vi "FarfiledImageJoint2.vi"() -> (1 "远场图像":T1(plugin-control))   [LabVIEW 2018]
uses:
  Init/AllPath.vi
  <vilib>/vision/NI_Vision_Development_Module.lvlib
panel:
  in  "停止":bool
  out "进度":dbl format="%05.2f%"
  out "俯仰":dbl
  out "Y Resolution":i32
  out "X Resolution":i32
  out "运行总时间s":dbl
  out "单步总时间ms":u32
  out "时间":u32[](array[numeric])
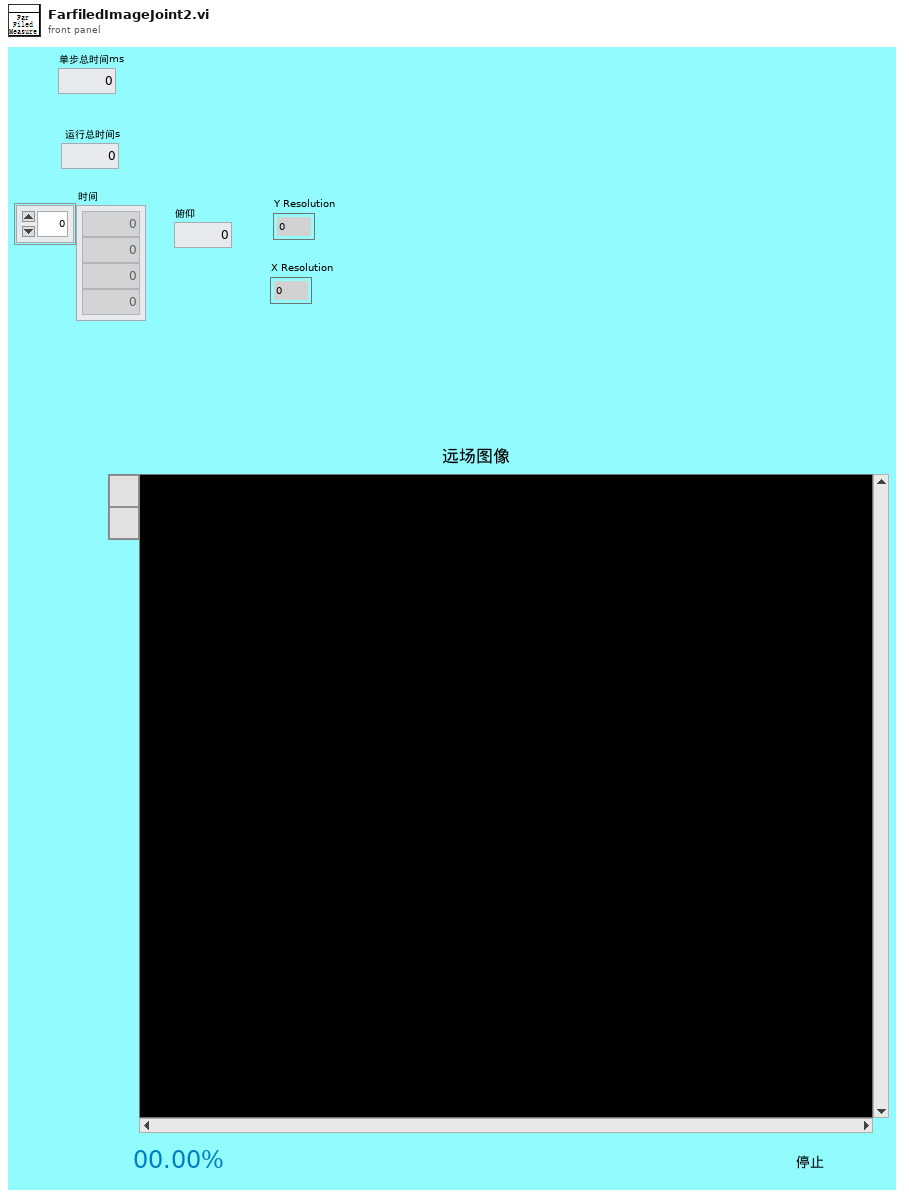
[diagram p1: front panel]
types:
  T1 = typedef "IMAQ Image.ctl" = refnum<image>
  T2 = typedef "Image Type" = u32
  T3 = typedef "控制电机枚举器.ctl" = enum16{"Z", "Y", "X", "发散角", "俯仰", "旋转"}
  T4 = cluster{"远场相机":cluster{"控制电机":T3, "位置":dbl}[], "近场相机":cluster{"控制电机":T3, "位置":dbl}[], "时间波形":cluster{"控制电机":T3, "位置":dbl}[], "偏振":cluster{"控制电机":T3, "位置":dbl}[], "能量":cluster{"控制电机":T3, "位置":dbl}[], "功率":cluster{"控制电机":T3, "位置":dbl}[], "光谱":cluster{"控制电机":T3, "位置":dbl}[], "准直光焦点":cluster{"控制电机":T3, "位置":dbl}[]}
  T5 = cluster{"能量/功率":path, " 示波器":path, " 光谱仪":path, "偏振":path, "近远场":cluster{" 近场图片":path, " 远场图片":path, "发散角数据":path}, "参数":path, " 基路径":path, "文件名信息":path, "输出模板路径":path, "输出报告路径":path}
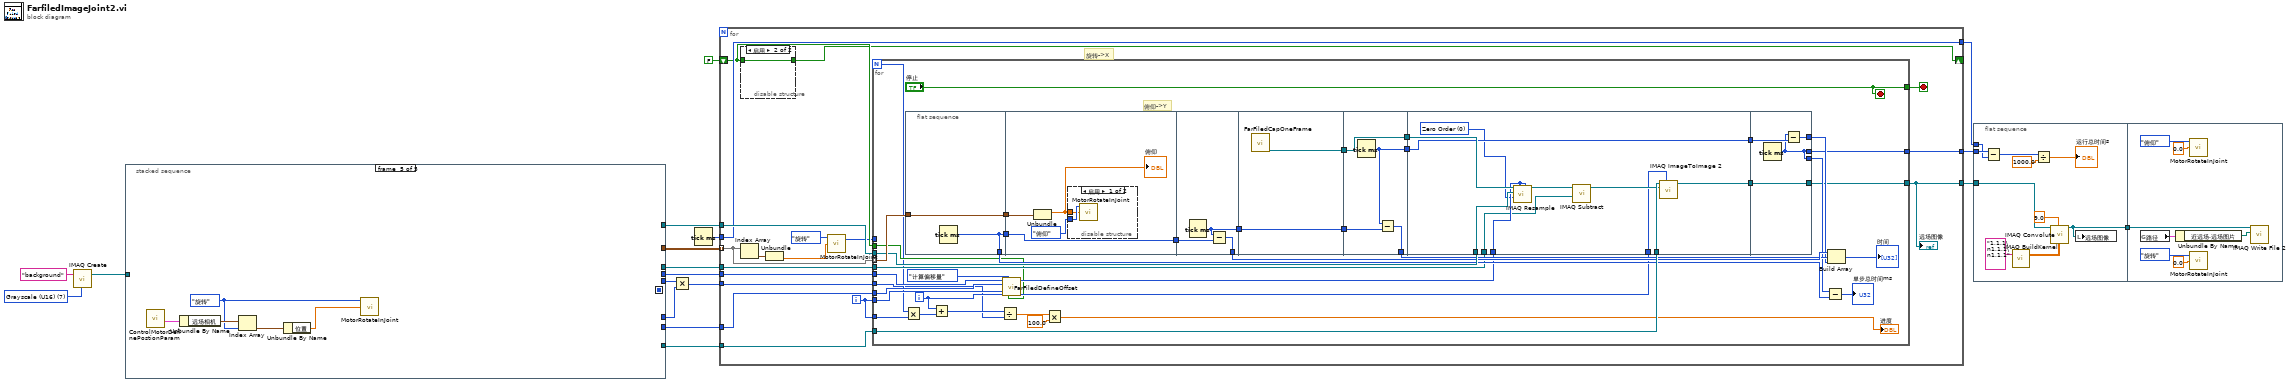
[diagram p0: block diagram]
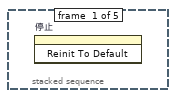
[diagram p2: hidden frame]
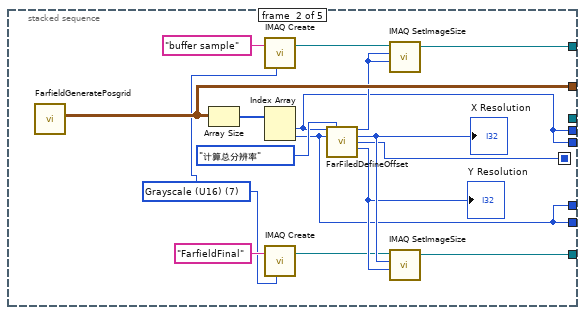
[diagram p3: hidden frame]
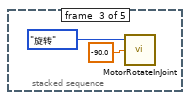
[diagram p4: hidden frame]
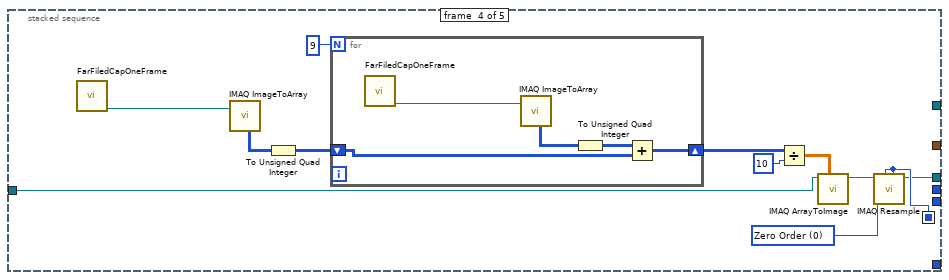
[diagram p5: hidden frame]
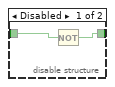
[diagram p6: hidden frame]
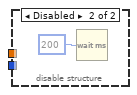
[diagram p7: hidden frame]
diagram:
  w1 = T2 7 items=["Grayscale (U8)", "Grayscale (I16)", "Grayscale (SGL)", "Complex (CSG)", "RGB (U32)", "HSL (U32)", "RGB (U64)", "Grayscale (U16)"] ("Image Type")
  n1 = call "IMAQ Create"("Image Name"="background", "Image Type"=w1) -> ("New Image"=w3:T1)  [unwired: 3 in, 1 out]
  n2 = stacked-sequence {
    seq-local: [_ w19 _ _ _] -> [_ _ _ w39 _]
    tunnel: [_ w34 _ _ _] -> w18
    tunnel: [_ w29 _ _ _] -> w17
    tunnel: [_ w28 _ _ _] -> w16
    tunnel: [_ w21 _ _ _] -> w15
    tunnel: [_ w22 _ _ _] -> w13
    tunnel: [_ _ _ w38 _] -> w9
    tunnel: [_ w22 _ _ _] -> w7
    tunnel: [_ w21 _ _ _] -> w6
    tunnel: w3 -> [_ _ _ w41 _]
    frame #0 {
      n3 = invoke on="停止" class="Bool" method="Reinit To Default"() -> ()  [unwired: 3 in, 3 out]
    }
    frame #1 {
      w26 = T2 7 items=["Grayscale (U8)", "Grayscale (I16)", "Grayscale (SGL)", "Complex (CSG)", "RGB (U32)", "HSL (U32)", "RGB (U64)", "Grayscale (U16)"] ("Image Type")
      n4 = call "FarfieldGeneratePosgrid.vi"() -> ("posOut"=w34:cluster{"俯仰":dbl, "旋转":dbl}[][])  [unwired: 9 in, 2 out]
      n5 = Array Size(array=w34) -> (size(s)=w33:i32[])
      n6 = call "IMAQ Create"("Image Name"="buffer sample", "Image Type"=w26) -> ("New Image"=w30:T1)  [unwired: 3 in, 1 out]
      n7 = Index Array(array=w33) -> (element #1=w22:i32, element #2=w21:i32)  [unwired: 2 in]
      n8 = call "IMAQ Create"("Image Name"="FarfieldFinal", "Image Type"=w26) -> ("New Image"=w20:T1)  [unwired: 3 in, 1 out]
      n9 = call "FarFiledDefineOffset.vi"("X Pos Num"=w22, "状态"=enum16{"计算总分辨率", "计算偏移量"}."计算总分辨率", "Y Pos Num"=w21) -> ("单个分辨率X"=w23:i32, "X Resolution"=w25:i32, "单个分辨率Y"=w19:i32, "Y Resolution"=w24:i32)  [unwired: 8 in, 1 out]
      "X Resolution" <- w25
      "Y Resolution" <- w24
      n10 = call "IMAQ SetImageSize"("Y Resolution"=w23, "X Resolution"=w23, "Image"=w30) -> ("Image Out"=w29:T1)  [unwired: 2 in, 1 out]
      n11 = call "IMAQ SetImageSize"("Y Resolution"=w24, "X Resolution"=w25, "Image"=w20) -> ("Image Out"=w28:T1)  [unwired: 2 in, 1 out]
    }
    frame #2 {
      n12 = call "MotorRotateInJoint.vi"("位置"=-90.0, "axis"=控制电机枚举器."旋转" ("控制电机")) -> ()  [unwired: 2 in, 1 out]
    }
    frame #3 {
      w37 = u32 0 items=["Zero Order", "Bi-Linear", "Quadratic", "Cubic Spline"] ("Interpolation Type")
      n13 = call "FarFiledCapOneFrame.vi"() -> ("Image_Normal"=w47:T1)  [unwired: 11 in]
      n14 = call "IMAQ ImageToArray"("Image"=w47) -> ("Image Pixels (U16)"=w45:u16[][])  [unwired: 3 in, 4 out]
      n15 = To Unsigned Quad Integer(1:w45) -> (0:w46:u64[][])
      n16 = for {
        N: 9 -> [_]
        shift-right: [w51] -> w44
        shift-left: w46 -> [w52]
        n17 = call "FarFiledCapOneFrame.vi"() -> ("Image_Normal"=w53:T1)  [unwired: 11 in]
        n18 = call "IMAQ ImageToArray"("Image"=w53) -> ("Image Pixels (U16)"=w50:u16[][])  [unwired: 3 in, 4 out]
        n19 = To Unsigned Quad Integer(1:w50) -> (0:w49:u64[][])
        n20 = Add(x=w49, y=w52) -> (x+y=w51:u64[][])
      }
      n21 = Divide(x=w44, y=10) -> (x/y=w42:dbl[][])
      n22 = call "IMAQ ArrayToImage"("Image Pixels (U16)"=w42, "Image"=w41) -> ("Image Out"=w40:T1)  [unwired: 8 in, 1 out]
      n23 = call "IMAQ Resample"("X Resolution"=w39, "Y Resolution"=w39, "Interpolation Type"=w37, "Image Src"=w40) -> ("Image Dst Out"=w38:T1)  [unwired: 6 in, 1 out]
    }
    frame #4 {
      w56 = 控制电机枚举器."旋转" ("控制电机")
      n24 = call "ControlMotorDefinePostionParam.vi"() -> ("位置信息"=w58:T4)  [unwired: 11 in]
      n25 = Unbundle By Name(w58) -> ("远场相机"=w57:cluster{"控制电机":T3, "位置":dbl}[])
      n26 = Index Array(array=w57, index=w56) -> (element=w55:cluster{"控制电机":T3, "位置":dbl})
      n27 = Unbundle By Name(w55) -> ("位置"=w54:dbl)
      n28 = call "MotorRotateInJoint.vi"("位置"=w54, "axis"=w56) -> ()  [unwired: 2 in, 1 out]
    }
  }
  n29 = Multiply(x=w7, y=w6) -> (x*y=w5:i32)
  n30 = Tick Count (ms)() -> (millisecond timer value=w12:u32)
  n31 = for "For循环" {
    tunnel: w18 -> [w72] mode=indexing
    tunnel: w17 -> [w76]
    tunnel: w13 -> [w74]
    tunnel: w15 -> [w73]
    shift-right: [w65] -> _
    shift-left: FALSE -> [w66]
    tunnel: w16 -> [w75]
    tunnel: [w62] -> w8
    tunnel: w12 -> [w67]
    tunnel: [w68] -> w11
    tunnel: [w67] -> w10
    tunnel: w9 -> [w64]
    tunnel: w5 -> [w59]
    i -> [w60]
    stop <- w61 stop-if-true
    # "旋转->X"
    n32 = disable-structure shown="启用" {
      disable-tunnel: w66 -> [w78 w79]
      disable-tunnel: [w77 w79] -> w65
      frame Disabled {
        n33 = Not(x=w78) -> (.not. x?=w77:bool)
      }
      frame Enabled {
      }
    }
    n34 = Index Array(array=w72) -> (element=w71:cluster{"俯仰":dbl, "旋转":dbl})  [unwired: 1 in]
    n35 = Unbundle(w71) -> ("旋转"=w69:dbl)  [unwired: 1 out]
    n36 = call "MotorRotateInJoint.vi"("位置"=w69, "axis"=控制电机枚举器."旋转" ("控制电机")) -> ("返回"=w63:i32)  [unwired: 2 in]
    n37 = for "For循环" {
      N -> [w84]
      tunnel: w72 -> [w119] mode=indexing
      tunnel: w76 -> [w118]
      tunnel: w60 -> [w97]
      tunnel: w74 -> [w95]
      tunnel: w73 -> [w96]
      tunnel: w66 -> [w92]
      tunnel: w75 -> [w117]
      tunnel: [w90] -> w62
      tunnel: [w100] -> w68
      tunnel: w64 -> [w99]
      tunnel: w63 -> [_]
      tunnel: ["停止"] -> w61
      tunnel: w60 -> [w85]
      tunnel: w59 -> [w83]
      i -> [w86]
      stop <- "停止" stop-if-true
      # "俯仰->Y"
      n38 = Multiply(x=w84, y=w85) -> (x*y=w88:i32)
      n39 = flat-sequence {
        tunnel: w119 -> [w121]
        tunnel: [w121] -> w112
        tunnel: [w120] -> w111
        tunnel: [w120] -> w102
        tunnel: w112 -> [w124]
        tunnel: w111 -> [w125]
        tunnel: [w125] -> w91
        tunnel: [w131] -> w110
        tunnel: w91 -> [w130]
        tunnel: [w129] -> w116
        tunnel: [w132] -> w109
        tunnel: w110 -> [w133]
        tunnel: [w133] -> w108
        tunnel: w109 -> [w137]
        tunnel: [w137] -> w107
        tunnel: [w135] -> w106
        tunnel: w108 -> [w136]
        tunnel: [w134] -> w115
        tunnel: w118 -> [w148]
        tunnel: w117 -> [w147]
        tunnel: w107 -> [w146]
        tunnel: w106 -> [w145]
        tunnel: [w141] -> w105
        tunnel: [w145] -> w104
        tunnel: w99 -> [w140]
        tunnel: w93 -> [w143]
        tunnel: w94 -> [w142]
        tunnel: [w152] -> w90
        tunnel: w105 -> [w152]
        tunnel: w104 -> [w151]
        tunnel: [w150] -> w114
        tunnel: [w149] -> w103
        tunnel: [w149] -> w100
        frame #0 {
          n40 = Tick Count (ms)() -> (millisecond timer value=w120:u32)
        }
        frame #1 {
          n41 = Unbundle(w124) -> ("俯仰"=w122:dbl)  [unwired: 1 out]
          "俯仰" <- w122
          n42 = disable-structure shown="启用" {
            disable-tunnel: 控制电机枚举器."俯仰" ("控制电机") -> [w127 _]
            disable-tunnel: w122 -> [w126 _]
            frame Enabled {
              n43 = call "MotorRotateInJoint.vi"("位置"=w126, "axis"=w127) -> ()  [unwired: 2 in, 1 out]
            }
            frame Disabled {
              n44 = Wait (ms)(milliseconds to wait=u32 200 ("等待时间（毫秒）")) -> ()  [unwired: 1 out]
            }
          }
        }
        frame #2 {
          n45 = Tick Count (ms)() -> (millisecond timer value=w131:u32)
          n46 = Subtract(x=w131, y=w130) -> (x-y=w129:u32)
        }
        frame #3 {
          n47 = call "FarFiledCapOneFrame.vi"() -> ("Image_Normal"=w132:T1)  [unwired: 11 in]
        }
        frame #4 {
          n48 = Tick Count (ms)() -> (millisecond timer value=w135:u32)
          n49 = Subtract(x=w135, y=w136) -> (x-y=w134:u32)
        }
        frame #5 {
          w139 = u32 0 items=["Zero Order", "Bi-Linear", "Quadratic", "Cubic Spline"] ("Interpolation Type")
          n50 = call "IMAQ Resample"("X Resolution"=w142, "Y Resolution"=w142, "Interpolation Type"=w139, "Image Dst"=w148, "Image Src"=w146) -> ("Image Dst Out"=w138:T1)  [unwired: 5 in, 1 out]
          n51 = call "IMAQ Subtract"("Image Src A"=w138, "Image Src B"=w140) -> ("Image Dst Out"=w144:T1)  [unwired: 5 in, 1 out]
          n52 = call "IMAQ ImageToImage 2"("Offset Left/Top"=w143, "Image Src (Small)"=w144, "Image Src (Large)"=w147) -> ("Image Dst Out"=w141:T1)  [unwired: 7 in, 1 out]
        }
        frame #6 {
          n53 = Tick Count (ms)() -> (millisecond timer value=w149:u32)
          n54 = Subtract(x=w149, y=w151) -> (x-y=w150:u32)
        }
      }
      n55 = Add(x=w86, y=w88) -> (x+y=w87:i32)
      n56 = Divide(x=w87, y=w83) -> (x/y=w82:dbl)
      n57 = call "FarFiledDefineOffset.vi"("X Pos Num"=w95, "状态"=enum16{"计算总分辨率", "计算偏移量"}."计算偏移量", "Y Pos Num"=w96, "当前X位置"=w97, "当前Y位置"=w86, "正序？"=w92) -> ("单个分辨率X"=w94:i32, "offset"=w93:i32[])  [unwired: 5 in, 3 out]
      n58 = Multiply(x=w82, y=100.0) -> (x*y=→"进度":dbl)
      n59 = Subtract(x=w103, y=w102) -> (x-y=→"单步总时间ms":u32)
      n60 = Build Array(w116, w115, w114) -> (→"时间":u32[])
    }
    "远场图像" <- w62
  }
  n61 = flat-sequence {
    tunnel: w11 -> [w162]
    tunnel: w10 -> [w161]
    tunnel: w8 -> [w154]
    tunnel: [w153] -> w4
    tunnel: w4 -> [w165]
    frame #0 {
      n62 = Subtract(x=w162, y=w161) -> (x-y=w160:u32)
      n63 = call "IMAQ BuildKernel"("Kernel String"="1,1,1\n1,1,1\n1,1,1") -> ("Kernel"=w155:sgl[][])  [unwired: 4 in, 1 out]
      n64 = Divide(x=w160, y=1000.0) -> (x/y=→"运行总时间s":dbl)
      n65 = call "IMAQ Convolute"("Kernel"=w155, "Divider (kernel sum)"=sgl 9.0, "Image Src"=w154) -> ("Image Dst Out"=w153:T1)  [unwired: 7 in, 1 out]
      n66 = local write "远场图像"(w153) -> ()
    }
    frame #1 {
      n67 = global read "AllPath.vi" "路径"() -> (w164:T5)
      n68 = Unbundle By Name(w164) -> ("近远场.远场图片"=w163:path)
      n69 = call "MotorRotateInJoint.vi"("位置"=0.0, "axis"=控制电机枚举器."俯仰" ("控制电机")) -> ()  [unwired: 2 in, 1 out]
      n70 = call "MotorRotateInJoint.vi"("位置"=0.0, "axis"=控制电机枚举器."旋转" ("控制电机")) -> ()  [unwired: 2 in, 1 out]
      n71 = call-poly "IMAQ Write File 2"("File Path"=w163, "Image"=w165) -> ()  [unwired: 8 in, 2 out]
    }
  }
